vi "iTacho_Find Complete Frame-setup.vi"(7 "test case ID":string) -> (2 "Read Buffer":string, 3 "iTacho":refnum<class "iTacho.lvclass">)   [LabVIEW 2018]
uses:
  Libraries/iTacho_class/iTacho.lvclass
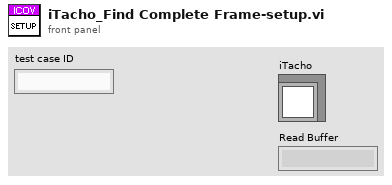
[diagram p1: front panel]
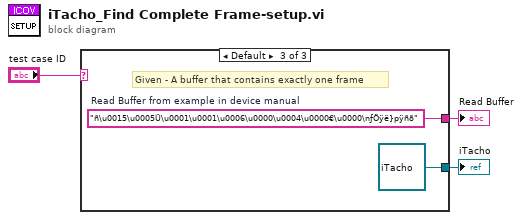
[diagram p0: block diagram]
diagram:
  n1 = case shown="Default" "test case ID" {
    tunnel: [_ _ w5] -> w2
    tunnel: [_ _ refnum<class "iTacho.lvclass"> refnum ("iTacho in")] -> w1
    frame "testcaseID1" {
    }
    frame "testcaseID2" {
    }
    frame Default {
      w5 = "ñ\u0015\u0005Ü\u0001\u0001\u0006\u0000\u0004\u0000€\u0000\nƒÖÿë}pÿñõ"  # Read Buffer from example in device manual
      # "Given - A buffer that contains exactly one frame"
    }
  }
  "Read Buffer" <- w2
  "iTacho" <- w1
